vi "Log Auto Data.vi"(11 "Record":bool) -> (3 "Done":bool)   [LabVIEW 2012]
uses:
  <vilib>/Utility/file.llb/Write To Spreadsheet File (DBL).vi
  Globals/Log Data.vi
panel:
  in  "file path":path=path "C:/AlexLog.txt"
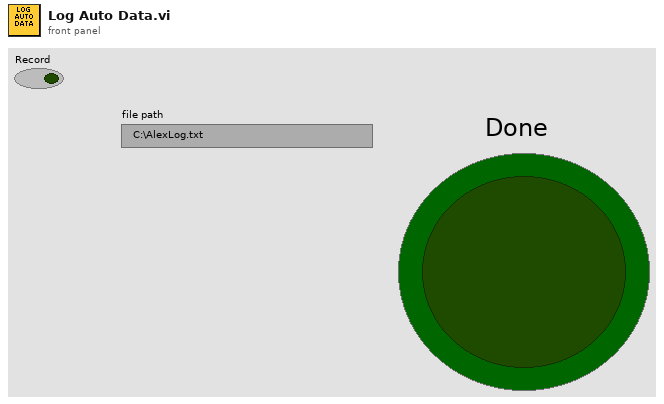
[diagram p1: front panel]
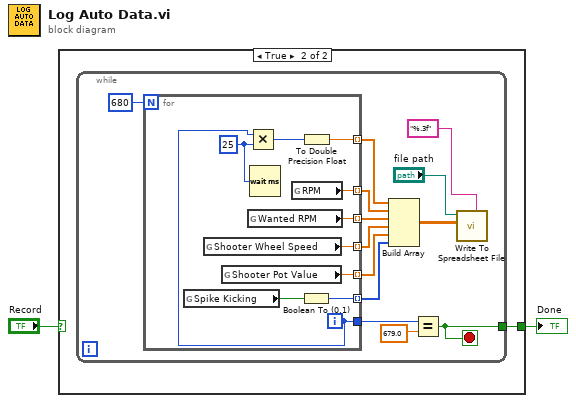
[diagram p0: block diagram]
diagram:
  n1 = case shown="True" "Record" {
    selector: "Record" -> [w3 _]
    tunnel: [w3 w4] -> w1
    frame False {
    }
    frame True {
      n2 = while {
        tunnel: [w11] -> w4
        stop <- w11 stop-if-true
        n3 = for {
          N: 680 -> [_]
          tunnel: [w18] -> w13
          tunnel: [w27] -> w10 mode=indexing
          tunnel: [w26] -> w9 mode=indexing
          tunnel: [w25] -> w8 mode=indexing
          tunnel: [w24] -> w7 mode=indexing
          tunnel: [w21] -> w6 mode=indexing
          tunnel: [w19] -> w5 mode=indexing
          i -> [w18]
          w23 = u32 25 ("milliseconds to wait")
          n4 = global read "Log Data.vi" "Spike Kicking"() -> (w20:bool)
          n5 = global read "Log Data.vi" "Shooter Wheel Speed"() -> (w25:dbl)
          n6 = global read "Log Data.vi" "Shooter Pot Value"() -> (w24:dbl)
          n7 = Multiply(x=w18, y=w23) -> (x*y=w22:u32)
          n8 = global read "Log Data.vi" "Wanted RPM"() -> (w26:dbl)
          n9 = Wait (ms)(milliseconds to wait=w23) -> ()  [unwired: 1 out]
          n10 = global read "Log Data.vi" "RPM"() -> (w27:dbl)
          n11 = Boolean To (0,1)(Boolean=w20) -> (0, 1=w19:i16)
          n12 = To Double Precision Float(number=w22) -> (double precision float=w21:dbl)
        }
        n13 = Build Array(w6, w10, w9, w8, w7, w5) -> (w15:dbl[][])
        n14 = Equal?(x=w13, y=679.0) -> (x = y?=w11:bool)
        n15 = call-poly <vilib>:"Write To Spreadsheet File.vi"("format (%.3f)"="%.3f", "2D data"=w15, "file path (dialog if empty)"="file path") -> ()  [unwired: 5 in, 1 out]
      }
    }
  }
  "Done" <- w1
